vi "CreatConnectOPC.vi"(10 "All Tags":string[](array[string]), 11 "URL":string="opc://localhost/National Instruments.NIOPCServers.V5/PA10.PA10 Laser Roigh Cutting._System") -> (3 "DsOut":T1[](array[typedef]))   [LabVIEW 2018]
uses:
  SubVIS.xio/DataSocket/DataSocket_Tags.ctl
  SubVIS.xio/DataSocket/Read PLC Vars/Read Bool Var.vi
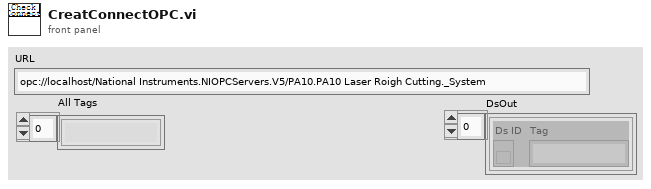
[diagram p1: front panel]
types:
  T1 = typedef "DataSocket_Tags.ctl" = cluster{"Ds ID":refnum<k13>, "Tag":string}
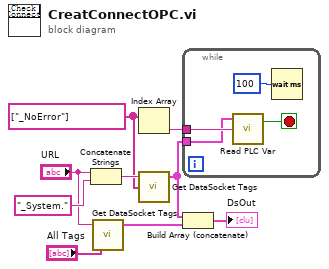
[diagram p0: block diagram]
diagram:
  w7 = string[] ["_NoError"] ("All Tags")
  n1 = Concatenate Strings("URL", "_System." ("字符串")) -> (w9:string)
  n2 = call "Get DataSocket Tags.vi"("All Tags"="All Tags", "URL"="URL") -> ("DsOut"=w4:T1[])  [unwired: 3 in]
  n3 = Index Array(array=w7) -> (element=w6:string)  [unwired: 1 in]
  n4 = call "Get DataSocket Tags.vi"("All Tags"=w7, "URL"=w9) -> ("DsOut"=w3:T1[])  [unwired: 3 in]
  n5 = while {
    tunnel: w6 -> [w11]
    tunnel: w3 -> [w10]
    stop <- w13 stop-if-true
    n6 = call-poly "Read PLC Var.vi"("Tag IN"=w11, "Ds PLCTags IN"=w10) -> ("Bool Var out"=w13:bool)  [unwired: 1 in, 1 out]
    n7 = Wait (ms)(milliseconds to wait=u32 100 ("等待时间（毫秒）")) -> ()  [unwired: 1 out]
  }
  n8 = Build Array (concatenate)(w3, w4) -> (→"DsOut":T1[])
